vi "Real Init.vi"(8 "error in (no error)":errorcluster, 11 "Local Error Manager in":refnum<class "Local Error Manager.lvclass">) -> (0 "error out":errorcluster, 3 "Local Error Manager out":refnum<class "Local Error Manager.lvclass">)   [LabVIEW 2020, in "TALOS.lvlib" / "Error Manager.lvlib" / "Local Error Manager.lvclass"]
uses:
  Local Error Manager.lvclass
  Local Error Manager.lvclass/Local Error Manager.ctl
  TALOS.lvlib
  Error Manager.lvclass
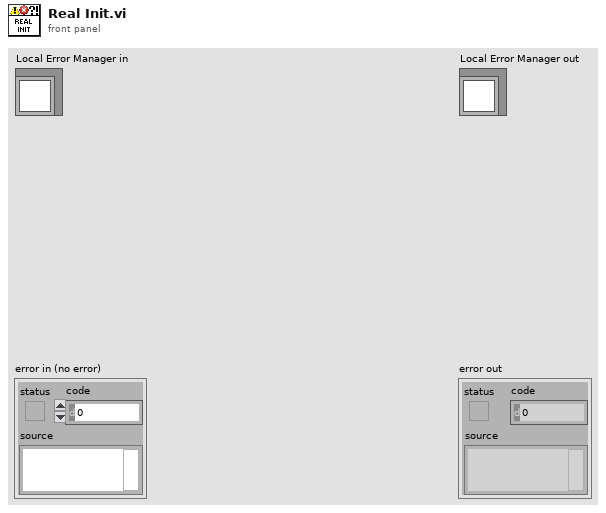
[diagram p1: front panel]
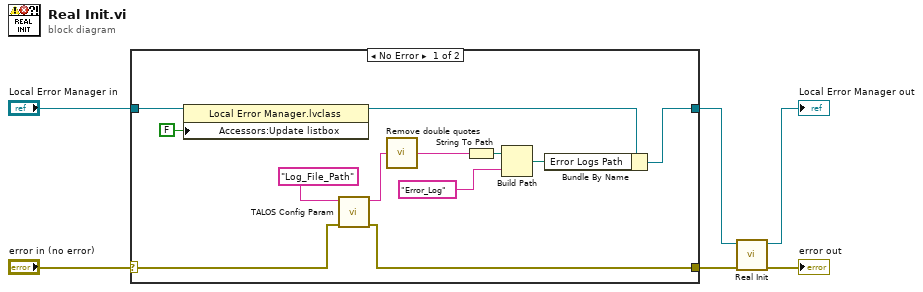
[diagram p0: block diagram]
diagram:
  n1 = case shown="No Error" "error in (no error)" {
    selector: "error in (no error)" -> [w13 w20]
    tunnel: [w12 w20] -> w4
    tunnel: [w10 w19] -> w2
    tunnel: "Local Error Manager in" -> [w11 w19]
    frame No Error {
      n2 = property class="Local Error Manager.lvclass"(reference=w11, "Accessors:Update listbox"=FALSE ("Update listbox")) -> (reference out=w8:refnum<class "Local Error Manager.lvclass">)  [unwired: 1 in, 1 out]
      n3 = call "TALOS Config Param.vi"("error in (no error)"=w13, "Parameter Name"="Log_File_Path") -> ("error out"=w12:errorcluster, "Output"=w15:string)  [unwired: 8 in]
      n4 = call "Remove double quotes.vi"("Input string"=w15) -> ("Output string"=w16:string)  [unwired: 4 in]
      n5 = String To Path(string=w16) -> (path=w17:path)
      n6 = Build Path(base path=w17, name or relative path="Error_Log") -> (appended path=w9:path)
      n7 = Bundle By Name(cluster=w8, "Error Logs Path"=w9) -> (w10:refnum<class "Local Error Manager.lvclass">)
    }
    frame Error {
    }
  }
  n8 = call-parent "Real Init.vi"("error in (no error)"=w4, "Error Manager in"=w2) -> ("error out"=→"error out":errorcluster, "Error Manager out"=→"Local Error Manager out":refnum<class "Local Error Manager.lvclass">)  [unwired: 8 in]
